vi "19052 Get_step_MODE.vi"(8 "error in (no error)":errorcluster, 9 "Step":u16=1 min=1 max=99 step=1, 11 "VISA resource in":refnum<visa-resource-name>) -> (0 "error out":errorcluster, 1 "Mode":string, 3 "VISA resource out":refnum<visa-resource-name>)   [LabVIEW 2015]
doc: "This VI obtains the mode of a selected step."
panel:
  out "output command":string
  # "Get step MODE"
  # "This is valid for both: \n19572 & 19052"
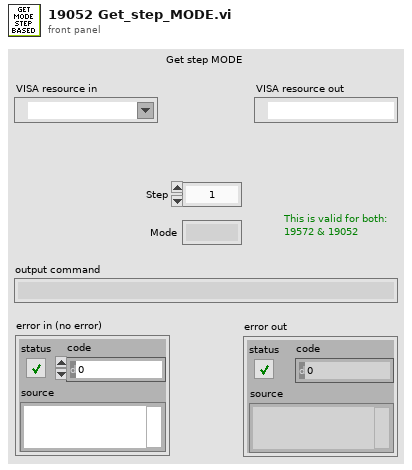
[diagram p1: front panel]
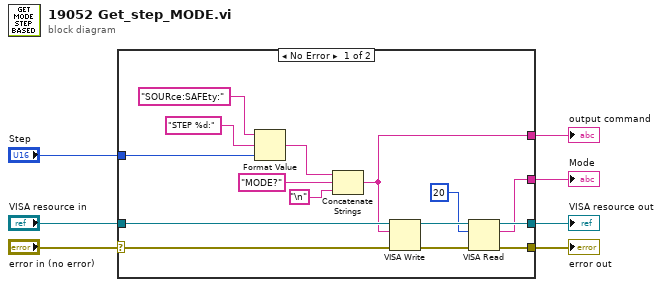
[diagram p0: block diagram]
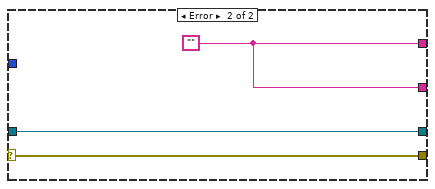
[diagram p2: hidden frame]
diagram:
  n1 = case shown="No Error" "error in (no error)" {
    selector: "error in (no error)" -> [w9 w24]
    tunnel: [w22 w24] -> w7
    tunnel: "VISA resource in" -> [w21 w25]
    tunnel: "Step" -> [w20 _]
    tunnel: [w15 w23] -> w5
    tunnel: [w11 w25] -> w4
    tunnel: [w10 w23] -> w3
    frame No Error {
      n2 = Format Value(string ("")="SOURce:SAFEty:", format string="STEP %d:", value (0)=w20) -> (output string=w8:string)
      n3 = Concatenate Strings(w8, "MODE?", "\n") -> (w15:string)
      n4 = VISA Write(VISA resource name=w21, write buffer=w15, error in (no error)=w9) -> (VISA resource name out=w13:refnum<visa-resource-name>, error out=w14:errorcluster)  [unwired: 1 out]
      n5 = VISA Read(VISA resource name=w13, byte count=u32 20, error in (no error)=w14) -> (VISA resource name out=w11:refnum<visa-resource-name>, read buffer=w10:string, error out=w22:errorcluster)  [unwired: 1 out]
    }
    frame Error {
      w23 = ""
    }
  }
  "error out" <- w7
  "VISA resource out" <- w4
  "output command" <- w5
  "Mode" <- w3
